vi "get data interface information.vi"(11 "fixed channel tag bus module in":refnum<class "fixed channel tag bus module.lvclass">) -> (2 "data type defs":T1, 3 "fixed channel tag bus module out":refnum<class "fixed channel tag bus module.lvclass">)   [LabVIEW 2013, in "fixed channel tag bus module.lvclass"]
uses:
  fixed channel tag bus module.lvclass
  fixed module parent/module/execution/data cluster type definition.ctl
  output user data.ctl
  parameter user data.ctl
  result user data.ctl
  input user data.ctl
  fixed module parent/module/execution/fixed channel runtime.lvclass
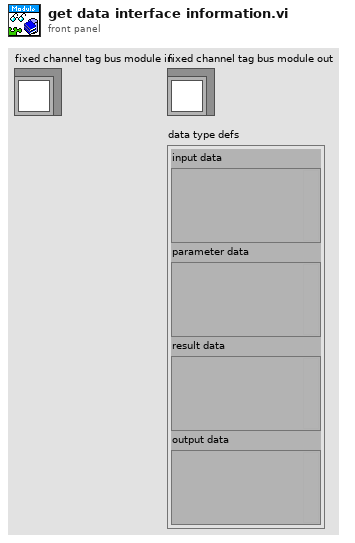
[diagram p1: front panel]
types:
  T1 = typedef "fixed channel runtime.lvclass/data cluster type definition.ctl" = cluster{"input data":variant, "parameter data":variant, "result data":variant, "output data":variant}
  T2 = typedef "fixed channel tag bus module.lvclass/input user data.ctl" = cluster{"placeholder":sgl}
  T3 = typedef "fixed channel tag bus module.lvclass/result user data.ctl" = cluster{"placeholder":sgl}
  T4 = typedef "fixed channel tag bus module.lvclass/parameter user data.ctl" = cluster{"placeholder":sgl}
  T5 = typedef "fixed channel tag bus module.lvclass/output user data.ctl" = cluster{"placeholder":sgl}
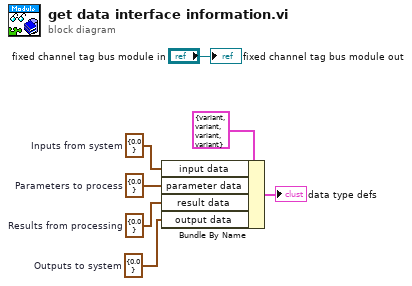
[diagram p0: block diagram]
diagram:
  w1 = T2 {"placeholder"=0.0}  # Inputs from system
  w3 = T3 {"placeholder"=0.0}  # Results from processing
  w2 = T4 {"placeholder"=0.0}  # Parameters to process
  w4 = T5 {"placeholder"=0.0}  # Outputs to system
  n1 = Bundle By Name(cluster=T1 {"input data"=variant, "parameter data"=variant, "result data"=variant, "output data"=variant} ("data type defs"), "input data"=w1, "parameter data"=w2, "result data"=w3, "output data"=w4) -> (→"data type defs":T1)
  "fixed channel tag bus module out" <- "fixed channel tag bus module in"
